vi "Add Alias.vi"(7 "Overwrite Existing?":bool=TRUE, 8 "error in (no error)":errorcluster, 9 "Alias Settings":T1, 10 "Base Node Path":string, 11 "SysDef Ref":T2) -> (0 "error out":errorcluster, 2 "New Node Path":string, 3 "SysDef Ref Out":T2)   [LabVIEW 2019, in "Simple SysDef API.lvlib"]
uses:
  <userlib>/SimpleSysDef/Simple SysDef API.lvlib
  <userlib>/SimpleSysDef/_SubVIs/System Definition Reference.ctl
  NationalInstruments.VeriStand.SystemDefinitionAPI
  <userlib>/SimpleSysDef/_SubVIs/Add Alias_Alias Settings.ctl
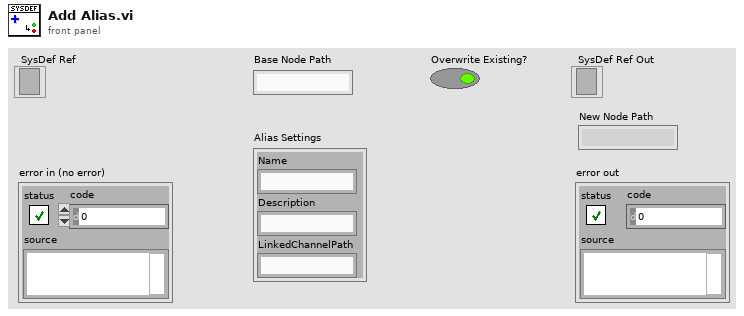
[diagram p1: front panel]
types:
  T1 = typedef "Simple SysDef API.lvlib/Add Alias_Alias Settings.ctl" = cluster{"Name":string, "Description":string, "LinkedChannelPath":string}
  T2 = typedef "Simple SysDef API.lvlib/System Definition Reference.ctl" = refnum<k24>
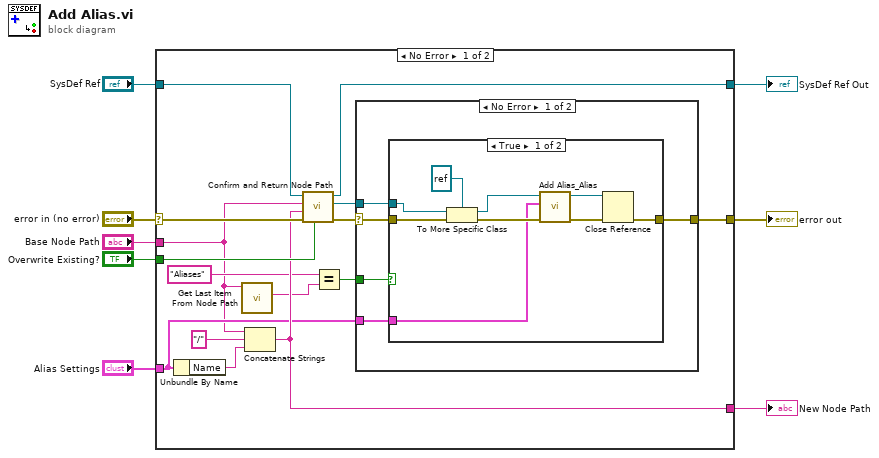
[diagram p0: block diagram]
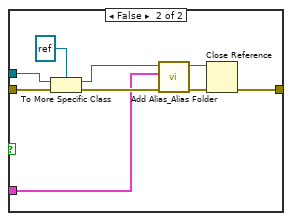
[diagram p2: hidden frame]
diagram:
  n1 = case shown="No Error" "error in (no error)" {
    selector: "error in (no error)" -> [w23 w49]
    tunnel: [w20 w49] -> w7
    tunnel: "SysDef Ref" -> [w22 w48]
    tunnel: [w9 w48] -> w5
    tunnel: "Base Node Path" -> [w11 _]
    tunnel: "Overwrite Existing?" -> [w17 _]
    tunnel: "Alias Settings" -> [w15 _]
    tunnel: [w16 _] -> w1
    frame No Error {
      n2 = Unbundle By Name(w15) -> ("Name"=w13:string)
      n3 = call <userlib>:"Get Last Item From Node Path.vi"("Name"=w11) -> ("Last Item"=w10:string)  [unwired: 9 in, 1 out]
      n4 = Concatenate Strings(w11, "/" ("string"), w13) -> (w16:string)
      n5 = call <userlib>:"Confirm and Return Node Path.vi"("Overwrite Existing?"=w17, "error in (no error)"=w23, "New Node Path"=w16, "Base Node Path"=w11, "SysDef Ref"=w22) -> ("error out"=w18:errorcluster, "Node Ref"=w19:refnum<k24>, "SysDef Ref Out"=w9:T2)  [unwired: 4 in]
      n6 = Equal?(x="Aliases", y=w10) -> (x = y?=w12:bool)
      n7 = case shown="No Error" w18 {
        selector: w18 -> [w27 w47]
        tunnel: [w26 w47] -> w20
        tunnel: w19 -> [w28 _]
        tunnel: w15 -> [w25 _]
        tunnel: w12 -> [w24 _]
        frame No Error {
          n8 = case shown="True" w24 {
            tunnel: w28 -> [w37 w46]
            tunnel: w27 -> [w29 w45]
            tunnel: [w36 w44] -> w26
            tunnel: w25 -> [w30 w38]
            frame True {
              n9 = To More Specific Class(target class=refnum<k24> refnum ("Node Ref"), reference=w37, error in=w29) -> (specific class reference=w31:refnum<k24>, error out=w33:errorcluster)
              n10 = call <userlib>:"Add Alias_Alias.vi"("error in (no error)"=w33, "Alias Settings"=w30, "Aliases Ref"=w31) -> ("error out"=w32:errorcluster, "Aliases Ref Out"=w34:refnum<k24>)  [unwired: 7 in]
              n11 = Close Reference(reference=w34, error in (no error)=w32) -> (error out=w36:errorcluster)
            }
            frame False {
              n12 = To More Specific Class(target class=refnum<k24> refnum ("Node Ref"), reference=w46, error in=w45) -> (specific class reference=w42:refnum<k24>, error out=w40:errorcluster)
              n13 = call <userlib>:"Add Alias_Alias Folder.vi"("error in (no error)"=w40, "Alias Settings"=w38, "Aliases Folder Ref"=w42) -> ("error out"=w39:errorcluster, "Aliases Folder Ref Out"=w41:refnum<k24>)  [unwired: 7 in]
              n14 = Close Reference(reference=w41, error in (no error)=w39) -> (error out=w44:errorcluster)
            }
          }
        }
        frame Error {
        }
      }
    }
    frame Error {
    }
  }
  "SysDef Ref Out" <- w5
  "error out" <- w7
  "New Node Path" <- w1
